vi "APS home move2.vi"(5 "ORG_Speed":i32, 6 "Max_Speed":i32, 7 "Start_Speed":i32, 8 "error in (no error)":errorcluster caption="错误输入（无错误）", 9 "Acc":i32, 10 "Dir":i32, 11 "Axis_ID":i32) -> (0 "error out":errorcluster caption="错误输出", 3 "function return":i32)   [LabVIEW 2011, in "APS168.lvlib"]
doc: "I32 FNTYPE APS_home_move2( I32 Axis_ID, I32 Dir, I32 Acc, I32 Start_Speed, I32 Max_Speed, I32 ORG_Speed );"
uses:
  APS168.lvlib
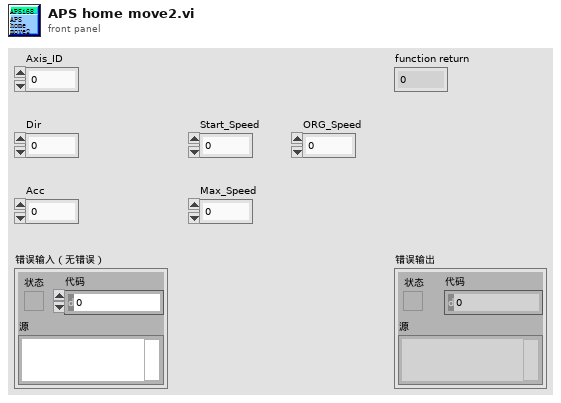
[diagram p1: front panel]
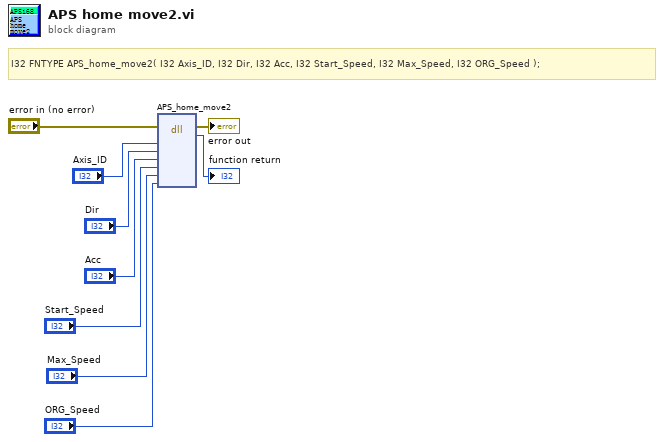
[diagram p0: block diagram]
diagram:
  # "I32 FNTYPE APS_home_move2( I32 Axis_ID, I32 Dir, I32 Acc, I32 Start_Speed, I32 Max_Speed, I32 ORG_Speed );"
  n1 = dll-call lib="PTH1Labs E软件ADLINK 204CAPS_1_7_1_LIB line 连续运动204APS168.*" fn="APS_home_move2"(error in="error in (no error)", "Axis_ID"="Axis_ID", "Dir"="Dir", "Acc"="Acc", "Start_Speed"="Start_Speed", "Max_Speed"="Max_Speed", "ORG_Speed"="ORG_Speed") -> (error out=→"error out":errorcluster, →"function return":i32)  [unwired: 8 in, 1 out]
